vi "Example tcp data collector.vi"() -> ()   [LabVIEW 2020]
uses:
  TCP subscription info cluster.ctl
panel:
  out "millisecond timer value":u32
  out "Requested values":string[](array[string])
  in  "TCP subscriptions info":T1
  in  "stop":bool
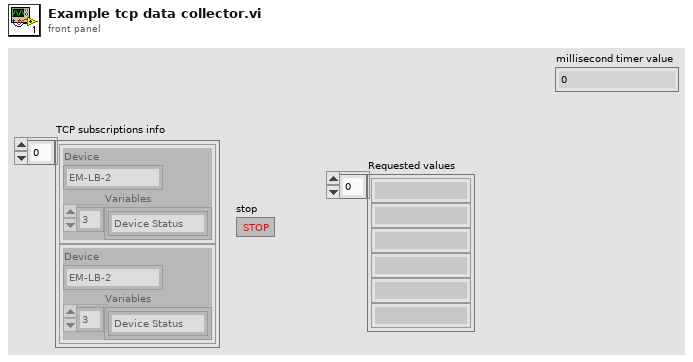
[diagram p1: front panel]
types:
  T1 = typedef "TCP subscription info cluster.ctl" = cluster{"Device":string, "Variables":string[]}[]
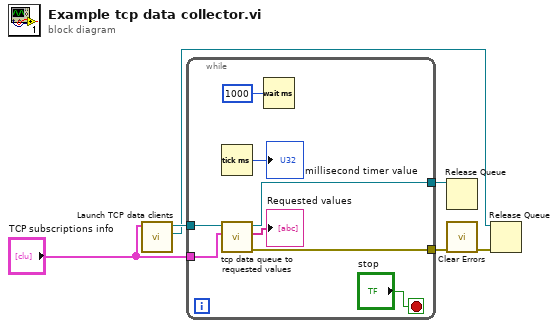
[diagram p0: block diagram]
diagram:
  n1 = call "Launch TCP data clients.vi"("TCP subscriptions info"="TCP subscriptions info") -> ("StopQueue"=w4:refnum<queue>, "DataQueue"=w6:refnum<queue>)  [unwired: 8 in, 1 out]
  n2 = while {
    tunnel: w6 -> [w13]
    tunnel: [w12] -> w5
    tunnel: [w11] -> w3
    tunnel: "TCP subscriptions info" -> [w8]
    stop <- "stop" stop-if-true
    n3 = Tick Count (ms)() -> (millisecond timer value=→"millisecond timer value":u32)
    n4 = call "tcp data queue to requested values.vi"("TCP subscriptions info"=w8, "Queue in"=w13) -> ("error out"=w11:errorcluster, "Array"=→"Requested values":string[], "Queue out"=w12:refnum<queue>)  [unwired: 7 in]
    n5 = Wait (ms)(milliseconds to wait=u32 1000) -> ()  [unwired: 1 out]
  }
  n6 = Release Queue(queue=w5) -> ()  [unwired: 2 in, 3 out]
  n7 = call <vilib>:"Clear Errors.vi"("error in (no error)"=w3) -> ("error out"=w2:errorcluster)  [unwired: 5 in, 1 out]
  n8 = Release Queue(queue=w4, error in (no error)=w2) -> ()  [unwired: 1 in, 3 out]
